vi "Ethernet Open.vi"(8 "error in (no error)":errorcluster, 10 "Ethernet Config":T1={"IP Address"=[192, 168, 0, 1], "Port No"=24691}, 11 "Device ID":i32) -> (0 "error out":errorcluster, 2 "Return Code":i32, 3 "Device ID out":i32)   [LabVIEW 2014, in "Keyence LJ-V7000.lvlib"]
uses:
  Keyence LJ-V7000.lvlib
  Clusters/Ethernet Config.ctl
panel:
  # "(c) 2012 KEYENCE CORPORATION.  ALL RIGHTS RESERVED."
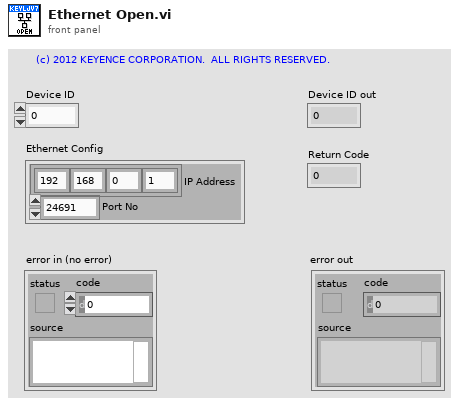
[diagram p1: front panel]
types:
  T1 = typedef "Keyence LJ-V7000.lvlib/Ethernet Config.ctl" = cluster{"IP Address":u8[], "Port No":u16}
  T2 = cluster{"IP Address[0]":u8, "IP Address[1]":u8, "IP Address[2]":u8, "IP Address[3]":u8}
  T3 = cluster{"IP Address":cluster{"IP Address[0]":u8, "IP Address[1]":u8, "IP Address[2]":u8, "IP Address[3]":u8}, "Port No":u16, "reserved":u8, "reserved":u8}
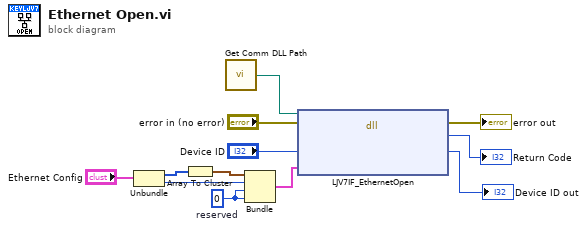
[diagram p0: block diagram]
diagram:
  w2 = u8 0  # reserved
  n1 = Unbundle("Ethernet Config") -> ("IP Address"=w5:u8[], "Port No"=w3:u16)
  n2 = Array To Cluster(array=w5) -> (cluster=w4:T2)
  n3 = call "Get Comm DLL Path.vi"() -> ("Comm DLL Path"=w7:path)  [unwired: 1 in]
  n4 = Bundle("IP Address"=w4, "Port No"=w3, "reserved"=w2, "reserved"=w2) -> (w1:T3)  [unwired: 1 in]
  n5 = dll-call lib="C:/Program Files/National Instruments/LabVIEW 2011/instr.lib/Keynece LJ-V7000/LJV7_IF.*" fn="LJV7IF_EthernetOpen"(path in=w7, error in="error in (no error)", "lDeviceId"="Device ID", "pEthernetConfig"=w1) -> (error out=→"error out":errorcluster, "lRetCode"=→"Return Code":i32, "lDeviceId"=→"Device ID out":i32)  [unwired: 2 in, 1 out]
